vi "Add VI Refnum to Destroy.vi"(8 "error in (no error)":errorcluster, 10 "key type":refnum<vi>, 11 "Async Methods Actor in":refnum<class "Async Methods Actor.lvclass">) -> (0 "error out":errorcluster, 3 "Async Methods Actor out":refnum<class "Async Methods Actor.lvclass">)   [LabVIEW 2021, in "Async Methods Actor.lvlib" / "Async Methods Actor.lvclass"]
uses:
  Async Methods Actor.lvclass
  Async Methods Actor.lvclass/Async Methods Actor.ctl
  <vilib>/ActorFramework/Actor/Actor.lvclass
  Async Methods Actor Messages/Async Message/Async Message.lvclass
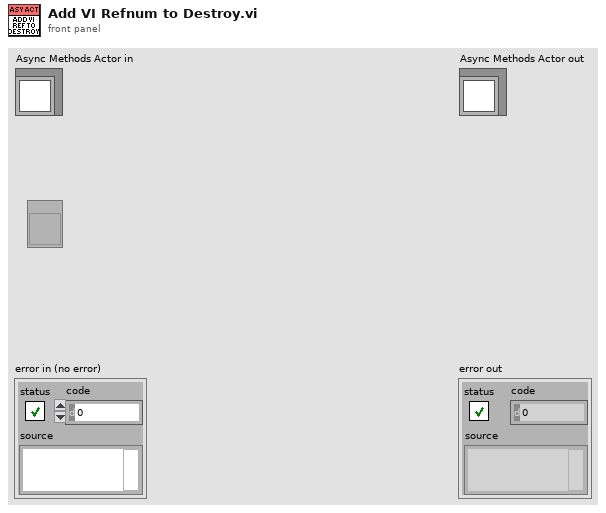
[diagram p1: front panel]
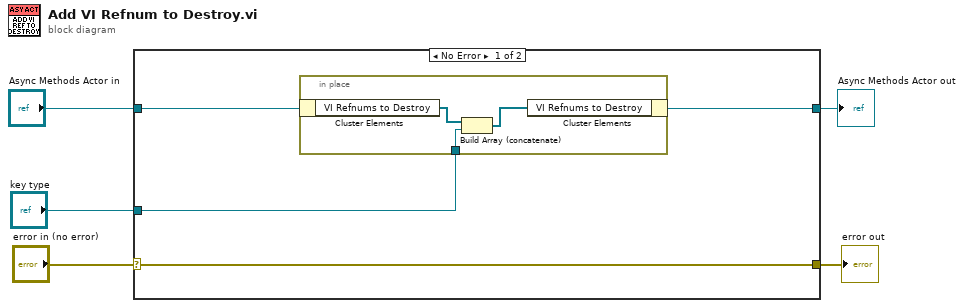
[diagram p0: block diagram]
diagram:
  n1 = case shown="No Error" "error in (no error)" {
    selector: "error in (no error)" -> [w8 w14]
    tunnel: [w8 w14] -> w4
    tunnel: [w7 w13] -> w2
    tunnel: "Async Methods Actor in" -> [w9 w13]
    tunnel: "key type" -> [w6 _]
    frame No Error {
      n2 = in-place {
        in-place-border: w6 -> [w10]
        n3 = in-place-cluster #1(w9) -> ("VI Refnums to Destroy"=w12:refnum<vi>[])
        n4 = Build Array (concatenate)(w12, w10) -> (w11:refnum<vi>[])
        n5 = in-place-cluster #1("VI Refnums to Destroy"=w11) -> (w7:refnum<class "Async Methods Actor.lvclass">)
      }
    }
    frame Error {
    }
  }
  "error out" <- w4
  "Async Methods Actor out" <- w2
